vi "Cal xy.vi"(0 "reference in":refnum<class "Mul.lvclass">, 5 "error in (no error)":errorcluster) -> (14 "reference out":refnum<class "Mul.lvclass">, 15 "result":dbl, 19 "error out":errorcluster)   [LabVIEW 2013, in "Mul.lvclass"]
uses:
  Mul.lvclass
  Operation_class/Operation.lvclass
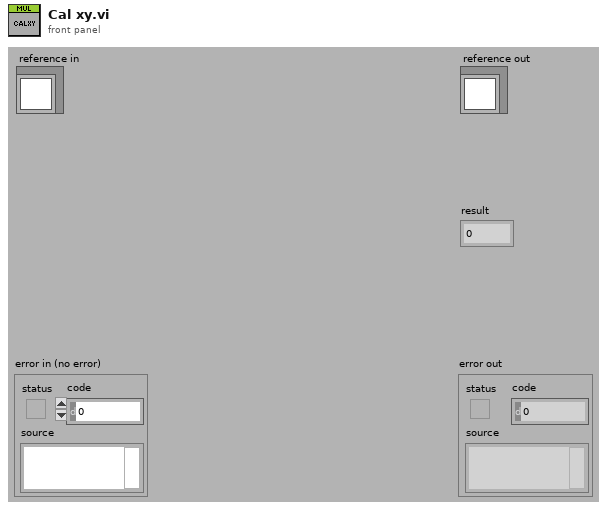
[diagram p1: front panel]
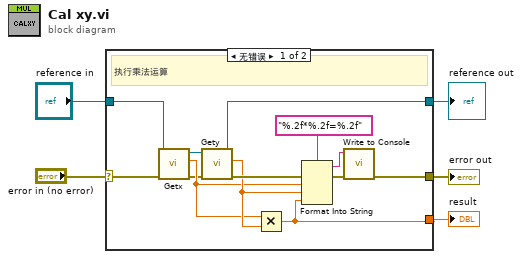
[diagram p0: block diagram]
diagram:
  n1 = case shown="无错误" "error in (no error)" {
    selector: "error in (no error)" -> [w11 w20]
    tunnel: [w7 w20] -> w4
    tunnel: [w9 w19] -> w2
    tunnel: "reference in" -> [w10 w19]
    tunnel: [w8 _] -> w1
    frame No Error {
      # "执行乘法运算"
      n2 = call "Getx.vi"("error in (no error)"=w11, "reference in"=w10) -> ("error out"=w13:errorcluster, "x"=w15:dbl, "reference out"=w12:refnum<class "Mul.lvclass">)  [unwired: 7 in]
      n3 = call "Gety.vi"("error in (no error)"=w13, "reference in"=w12) -> ("error out"=w18:errorcluster, "y"=w16:dbl, "reference out"=w9:refnum<class "Mul.lvclass">)  [unwired: 7 in]
      n4 = Multiply(x=w15, y=w16) -> (x*y=w8:dbl)
      n5 = Format Into String(format string="%.2f*%.2f=%.2f" ("格式字符串"), error in=w18, w15, w16, w8) -> (resulting string=w6:string, error out=w17:errorcluster)  [unwired: 1 in]
      n6 = call "Write to Console.vi"("error in (no error)"=w17, "Input"=w6) -> ("error out"=w7:errorcluster)  [unwired: 9 in]
    }
    frame Error {
    }
  }
  "error out" <- w4
  "reference out" <- w2
  "result" <- w1
